vi "Tree.vi"   [LabVIEW 2016, in "DemoSkeleton.lvlib"]
uses:
  DemoSkeleton.lvlib
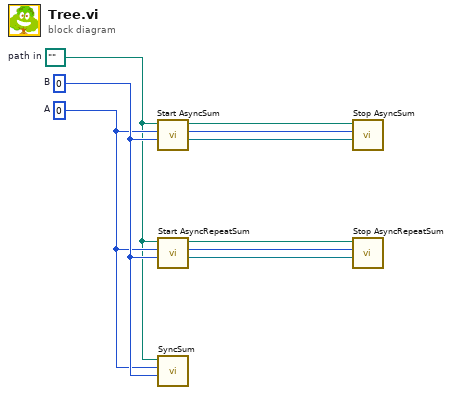
[diagram p0: block diagram]
diagram:
  w3 = path ""  # path in
  w5 = 0  # B
  w4 = 0  # A
  n1 = call "Start AsyncSum.vi"("B"=w5, "A"=w4, "path in"=w3) -> ("LVUserEvent CallBack Reference"=w2:refnum<user-event>, "Handle"=w8:u64, "dup path"=w9:path)  [unwired: 4 in, 2 out]
  n2 = call "Start AsyncRepeatSum.vi"("B"=w5, "A"=w4, "path in"=w3) -> ("LVUserEvent CallBack Reference"=w1:refnum<user-event>, "Handle"=w6:u64, "dup path"=w7:path)  [unwired: 4 in, 2 out]
  n3 = call "SyncSum.vi"("B"=w5, "A"=w4, "path in"=w3) -> ()  [unwired: 6 in, 3 out]
  n4 = call "Stop AsyncSum.vi"("LVUserEventCallBackRef"=w2, "Handle"=w8, "path in"=w9) -> ()  [unwired: 7 in, 2 out]
  n5 = call "Stop AsyncRepeatSum.vi"("LVUserEventCallBackRef"=w1, "Handle"=w6, "path in"=w7) -> ()  [unwired: 7 in, 2 out]
